vi "周期测量_大范围.vi"() -> ()   [LabVIEW 2013]
doc: "This example demonstrates how to count the pulse's edges."
uses:
  <userlib>/ArtDAQ/_SubVI/ArtDAQ_CreateCIPeriodChan.vi
  <userlib>/ArtDAQ/_SubVI/ArtDAQ_CfgImplicitTiming.vi
  <userlib>/ArtDAQ/_SubVI/ArtDAQ_Read Counter DBL NSamp.vi
panel:
  in  "除数":u32=4
  in  "开始边沿":i32(ring)=10280 items=["上升"=10280, "下降"=10171]
  out "数据":dbl[](array[numeric])
  in  "每通道点数":i32=10
  in  "计时器":string="Dev2/Ctr0"
  in  "最小值":dbl=1e-06 format="%0.6f"
  in  "最大值":dbl=10.0 format="%0.6f"
  in  "Stop":bool
  out "错误输出":errorcluster
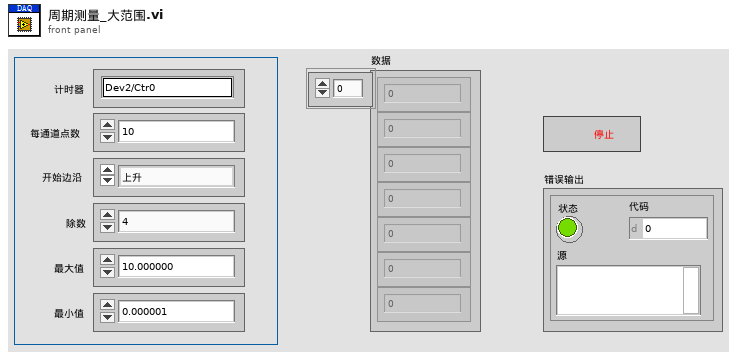
[diagram p1: front panel]
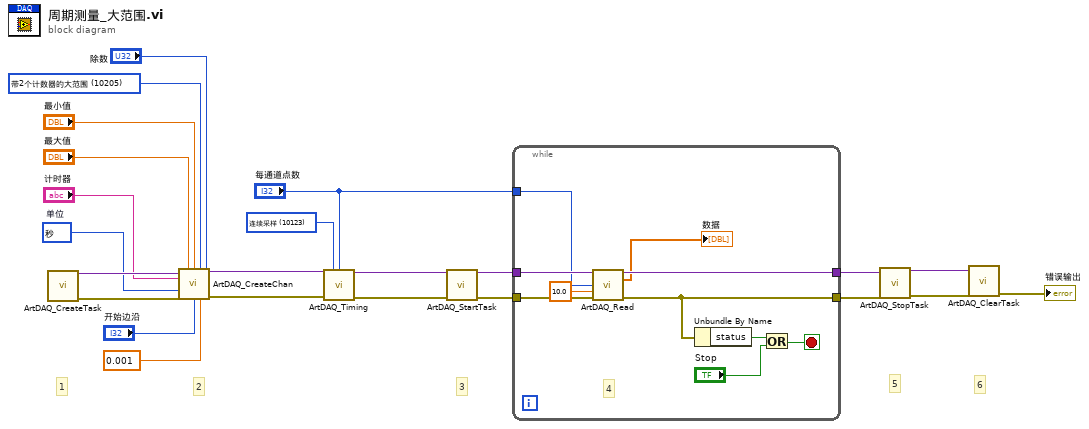
[diagram p0: block diagram]
diagram:
  w4 = 10364 items=["秒"=10364, "时钟滴答"=10304, "来自自定义换算"=10065]  # 单位
  w6 = 10205 items=["带1个计数器的低频"=10105, "带2个计数器的高频"=10157, "带2个计数器的大范围"=10205] ("测量方法")
  w7 = 10123 items=["有限点采样"=10178, "连续采样"=10123] ("采样模式")
  # "6"
  # "5"
  # "3"
  # "2"
  # "1"
  n1 = call <userlib>:"ArtDAQ_CreateTask.vi"() -> ("任务句柄"=w23:variant, "错误输出"=w22:errorcluster)  [unwired: 14 in]
  n2 = call-poly <userlib>:"ArtDAQ_CreateChan.vi"("任务句柄"=w23, "最大值"="最大值", "最小值"="最小值", "测量方法"=w6, "计数器"="计时器", "除数"="除数", "单位"=w4, "错误输入"=w22, "开始边沿"="开始边沿", "测量时间"=0.001) -> ("任务句柄"=w11:variant, "错误输出"=w8:errorcluster)  [unwired: 4 in]
  n3 = call-poly <userlib>:"ArtDAQ_Timing.vi"("任务句柄"=w11, "采样模式"=w7, "每通道采样数"="每通道点数", "错误输入"=w8) -> ("任务句柄"=w10:variant, "错误输出"=w9:errorcluster)  [unwired: 10 in]
  n4 = call <userlib>:"ArtDAQ_StartTask.vi"("任务句柄"=w10, "错误输入"=w9) -> ("任务句柄"=w15:variant, "错误输出"=w14:errorcluster)  [unwired: 12 in]
  n5 = while {
    tunnel: [w33] -> w20
    tunnel: [w29] -> w18
    tunnel: w15 -> [w32]
    tunnel: w14 -> [w31]
    tunnel: "每通道点数" -> [w25]
    stop <- w26 stop-if-true
    # "4"
    n6 = call-poly <userlib>:"ArtDAQ_Read.vi"("任务句柄"=w32, "每通道采样数"=w25, "超时s"=10.0 ("Timeout"), "错误输入"=w31) -> ("任务句柄"=w33:variant, "数据"=→"数据":dbl[], "错误输出"=w29:errorcluster)  [unwired: 8 in, 1 out]
    n7 = Unbundle By Name(w29) -> ("status"=w28:bool)
    n8 = Or(x=w28, y="Stop") -> (x .or. y?=w26:bool)
  }
  n9 = call <userlib>:"ArtDAQ_StopTask.vi"("任务句柄"=w20, "错误输入"=w18) -> ("任务句柄"=w19:variant, "错误输出"=w17:errorcluster)  [unwired: 12 in]
  n10 = call <userlib>:"ArtDAQ_ClearTask.vi"("任务句柄"=w19, "错误输入"=w17) -> ("错误输出"=→"错误输出":errorcluster)  [unwired: 13 in]
